vi "Async.vi"() -> ()   [LabVIEW 2012, in "Waveform Data Logger Engine.lvlib"]
uses:
  Waveform Data Logger Engine.lvlib
  Types/RT Data.ctl
  <vilib>/NI Veristand/Custom Device API/Custom Device Item Ref.ctl
  Types/Inline Waveform Info.ctl
  <vilib>/NI Veristand/Custom Device API/Waveform Data Reference.ctl
  Classes/Waveforms/Waveform Receive/Associated Log.ctl
  <vilib>/NI Veristand/Custom Device API/Custom Device Waveform DataType.ctl
  Types/Channels.ctl
  <vilib>/NI Veristand/Custom Device API/Block Data Reference.ctl
  <vilib>/NI Veristand/Custom Device API/Data Reference.ctl
  Types/System Time.ctl
  Types/Inline Waveform Log Info.ctl
  Shared/Classes/Log File Specifications/Waveform TDMS Log File Specification/Waveform TDMS Log File Specification.lvclass
  Classes/Triggers/Trigger/Trigger.lvclass
  Types/Inline Log Waveform.ctl
  Types/Trigger Settings.ctl
  Types/Log Status.ctl
  Types/Channel.ctl
  Types/Communication.ctl
  Types/Async Status.ctl
  Types/Async State.ctl
  <vilib>/NI Veristand/Custom Device Waveform API/Communication Properties.ctl
  Types/Trigger Event Data.ctl
  Types/Trigger Received.ctl
  Types/New File Event Data.ctl
  Types/Log Queues.ctl
  <vilib>/NI Veristand/Custom Device Waveform API/Waveform Session.lvclass/Waveform Session.ctl
  <vilib>/NI Veristand/Custom Device Waveform API/Multiple Waveforms Read (DBL)/Multiple Waveforms Read (DBL).lvclass/Multiple Waveforms Read (DBL).ctl
  <vilib>/NI Veristand/Custom Device Waveform API/Internal Comm Classes/WPL Comm/WPL Comm (1D DBL)/WPL Comm (1D DBL).lvclass/WPL Comm (1D DBL).ctl
  Classes/Waveforms/Utilities/Reference Dictionary/Reference Dictionary.lvclass/Reference Dictionary.ctl
  Classes/Waveforms/Waveform Receive/Waveform Receive.lvclass/Waveform Receive.ctl
  Classes/Waveforms/Waveform Log/Waveform Log.lvclass/Waveform Log.ctl
  Classes/Logs/Segmented Logs/Segmented Log/Segmented Log.lvclass/Segmented Log.ctl
  Shared/Classes/Log File Specifications/Log File Specification/Log File Specification.lvclass/Log File Specification.ctl
  Shared/Classes/Log File Specifications/Waveform TDMS Log File Specification/Waveform TDMS Log File Specification.lvclass/Waveform TDMS Log File Specification.ctl
  Classes/Logs/Log Files/Log File/Log File.lvclass/Log File.ctl
  Classes/Logs/Log Files/TDMS Log File/TDMS Log File.lvclass/TDMS Log File.ctl
  Classes/Logs/Log Files/Text Log File/Text Log File.lvclass/Text Log File.ctl
  Classes/Logs/Segmented Logs/Footprint Segmented Log/Footprint Segmented Log.lvclass/Footprint Segmented Log.ctl
  Classes/Logs/Segmented Logs/Time Segmented Log/Time Segmented Log.lvclass/Time Segmented Log.ctl
  Classes/Waveforms/Buffer/Waveform Buffer/Waveform Buffer.lvclass/Waveform Buffer.ctl
  Classes/Waveforms/Buffer/DBL Waveform Buffer/DBL Waveform Buffer.lvclass/DBL Waveform Buffer.ctl
  Types/Check File Loop Cmd.ctl
  <vilib>/NI Veristand/Custom Device Waveform API/NI VeriStand - Read Waveform(s).vi
  <vilib>/NI Veristand/Custom Device Waveform API/Multiple Waveforms Read (DBL)/NI VeriStand - Read Multiple Waveforms (DBL).vi
  Classes/Waveforms/Utilities/Reference Dictionary/Lookup (Wfm Data Ref).vi
  Classes/Waveforms/Waveform Log/Write Current Waveform to Log Instances.vi
  Classes/Waveforms/Waveform Log/Update Missed Samples.vi
  Classes/Waveforms/Waveform Receive/Check Missed Samples.vi
  Classes/Waveforms/Buffer/Waveform Buffer/Write Waveform to Buffer (DBL).vi
  Classes/Waveforms/Buffer/Waveform Buffer/Set dt.vi
  Classes/Waveforms/Waveform Receive/Get dt.vi
  Classes/Waveforms/Waveform Receive/Check For DBL Equality.vi
  Classes/Waveforms/Buffer/Waveform Buffer/Get Segments in Range.vi
  Classes/Waveforms/Buffer/Waveform Buffer/Read Waveform Segment (DBL).vi
  Classes/Waveforms/Waveform Log/Write to Waveform Log Instance.vi
  Classes/Waveforms/Waveform Log/Update Log Status.vi
  <vilib>/NI Veristand/Custom Device Waveform API/Internal Comm Classes/WPL Comm/WPL Comm (1D DBL)/Comm_read 1d dbl.vi
  <vilib>/NI Veristand/Custom Device Waveform API/Check Opened.vi
  Classes/Waveforms/Waveform Log/Get Waveform In Range.vi
  Classes/Waveforms/Buffer/DBL Waveform Buffer/DBL Write to Buffer.vi
  Classes/Waveforms/Buffer/Waveform Buffer/Update Current Segment.vi
  Classes/Waveforms/Buffer/Waveform Buffer/Check New Segment.vi
  Classes/Waveforms/Buffer/Waveform Buffer/Update Waveform Segments.vi
  Classes/Waveforms/Buffer/Waveform Buffer/Resize Buffer.vi
  Classes/Waveforms/Buffer/Waveform Buffer/Shift Point by Time.vi
  Classes/Waveforms/Buffer/Waveform Buffer/Split Divided Segment.vi
  Classes/Waveforms/Buffer/DBL Waveform Buffer/DBL Read from Buffer.vi
  Classes/Logs/Segmented Logs/Segmented Log/Write Waveform to Log File Instance.vi
  <vilib>/NI Veristand/Custom Device Waveform API/Internal Comm Classes/WPL Comm/Convert Q Error to Shutdown Error.vi
  Classes/Waveforms/Buffer/Waveform Buffer/Get Current Buffer Index.vi
  Classes/Waveforms/Buffer/Waveform Buffer/Get Buffer Length.vi
  Classes/Waveforms/Buffer/Waveform Buffer/Shift Point by Samples.vi
  Classes/Waveforms/Buffer/DBL Waveform Buffer/DBL Resize Buffer.vi
  Shared/Classes/Log File Specifications/Log File Specification/Get Log Specification Type.vi
  Shared/Classes/Log File Specifications/Waveform TDMS Log File Specification/Get Current Group.vi
  Classes/Logs/Log Files/Log File/Get Log File Type.vi
  Classes/Logs/Log Files/Log File/Write Channel to Log File.vi
  Classes/Logs/Log Files/TDMS Log File/Set TDMS Channel Property.vi
  Classes/Logs/Log Files/TDMS Log File/Copy Channel Properties.vi
  Classes/Logs/Segmented Logs/Segmented Log/Check Close File.vi
  Classes/Logs/Segmented Logs/Segmented Log/Check Open File.vi
  Classes/Logs/Log Files/TDMS Log File/Write Channel to TDMS Log File.vi
  Classes/Logs/Log Files/Text Log File/Write Channel to Text Log File.vi
  Classes/Logs/Segmented Logs/Segmented Log/Close Log File Instance.vi
  Classes/Logs/Segmented Logs/Segmented Log/Segment Log File.vi
  Classes/Logs/Segmented Logs/Segmented Log/Open Log File Instance.vi
  Classes/Logs/Log Files/Log File/Close Log File.vi
  Classes/Logs/Segmented Logs/Segmented Log/Make File Read-Only.vi
  Classes/Logs/Segmented Logs/Segmented Log/On Segmented Log Complete.vi
  Classes/Logs/Segmented Logs/Segmented Log/On File Close.vi
  Classes/Logs/Segmented Logs/Footprint Segmented Log/Segment Log File (Footprint).vi
  Classes/Logs/Segmented Logs/Time Segmented Log/Segment Log File (Time).vi
  Shared/Classes/Log File Specifications/Log File Specification/Open Log File.vi
  Shared/Classes/Log File Specifications/Log File Specification/Set Path Tag.vi
  Classes/Logs/Segmented Logs/Segmented Log/On File Open.vi
  Shared/Classes/Log File Specifications/Log File Specification/Set Filename Offset.vi
  Classes/Logs/Log Files/TDMS Log File/Close TDMS Log File.vi
  Classes/Logs/Log Files/Text Log File/Close Text Log File.vi
  Classes/Logs/Segmented Logs/Segmented Log/Get Current Log File Instance.vi
  Classes/Logs/Log Files/Log File/Get File Size.vi
  Classes/Logs/Log Files/Log File/Get Start Time.vi
  Shared/Classes/Log File Specifications/Log File Specification/Build File Path.vi
  Shared/Classes/Log File Specifications/Log File Specification/Resolve File Conflicts.vi
  <vilib>/Utility/error.llb/Error Cluster From Error Code.vi
  Classes/Waveforms/Waveform Log/Check Instance Done.vi
  Shared/Classes/Log File Specifications/Log File Specification/Initialize Log File.vi
  <vilib>/Utility/libraryn.llb/Check if File or Folder Exists.vi
  <vilib>/Utility/libraryn.llb/Get File Extension.vi
  <vilib>/Utility/libraryn.llb/Create Directory Recursive.vi
  <userlib>/_OpenG.lib/error/error.llb/Filter Error Codes (Array)__ogtk.vi
  <vilib>/NI Veristand/Custom Device Tools/Custom Device Utility Library/NI VeriStand - Print Debug String.vi
  <vilib>/Utility/error.llb/Simple Error Handler.vi
  Classes/Waveforms/Waveform Receive/Waveform Receive.lvclass
  Classes/Logs/Log Files/Log File/Log File.lvclass
  Classes/Logs/Log Files/TDMS Log File/TDMS Log File.lvclass
  Classes/Logs/Log Files/Text Log File/Text Log File.lvclass
  Classes/Logs/Segmented Logs/Footprint Segmented Log/Footprint Segmented Log.lvclass
  Classes/Logs/Segmented Logs/Time Segmented Log/Time Segmented Log.lvclass
  Classes/Waveforms/Buffer/DBL Waveform Buffer/DBL Waveform Buffer.lvclass
  Classes/Waveforms/Buffer/CDB Waveform Buffer/CDB Waveform Buffer.lvclass
  <vilib>/NI VeriStand/Custom Device Waveform API/NI_VS Custom Device Waveform API.lvlib
  Classes/Waveforms/Waveform Log/Waveform Log.lvclass
  <vilib>/NI Veristand/Custom Device Waveform API/Multiple Waveforms Read (CDB)/NI VeriStand - Open Multiple Waveforms Read Session (CDB).vi
  <vilib>/NI Veristand/Custom Device Waveform API/Multiple Waveforms Read (CDB)/Multiple Waveforms Read (CDB).lvclass
  <vilib>/NI Veristand/Custom Device API/Custom Device API.lvlib
panel:
  in  "Async Input":T1={"Device Ref"=18446744073709551615, "Waveforms"=[], "Channels"={"Command Chan Refs"=[], "Command Data Refs"=[], "Command Values"=[], "Status Chan Refs"=[], "Status Data Refs"=[], "Status Values"=[], "System Time"={"System Time"=timestamp(0 s since 1904-01-01), "Data Reference"=0, "Absolute Time Channel Data Ref"=0, "Get Date-Time Channel Data Ref"=0}, "Trigger Chan Refs"=[], "Trigger Data Refs"=[], "Trigger Values"=[]}, "Waveform Logs"=[], "Communication"={"Async Status"=refnum, "Wfm Comm Properties"={"WPL"={"Custom Queue Size"=1, "Use Custom Queue Size?"=FALSE}}, "Shutdown Event"=refnum, "Trigger Event"=refnum, "New File Event"=refnum, "Log Queues"=[], "Async VI Ref"=refnum}, "error"={"status"=FALSE, "code"=0, "source"=""}} {"Device Ref" format="%.0x"; "Channels"."Trigger Data Refs"."Data Reference" format="%.0x"; "Channels"."Trigger Chan Refs" format="%.0x"; "Channels"."System Time"."Get Date-Time Channel Data Ref" format="%.0x"; "Channels"."System Time"."Absolute Time Channel Data Ref" format="%.0x"; "Channels"."System Time"."Channel Data Reference" format="%.0x"; "Channels"."Status Data Refs"."Data Reference" format="%.0x"; "Channels"."Command Data Refs"."Data Reference" format="%.0x"; "Channels"."Status Chan Refs" format="%.0x"; "Channels"."Command Chan Refs" format="%.0x"; "Waveforms"."Waveform Ref in" format="%.0x"; "Waveform Logs"."Node ID" format="%.0x"; "Waveform Logs"."TDMS Error Code"."Data Ref" format="%.0x"; "Waveform Logs"."Missed Samples"."Data Ref" format="%.0x"; "Waveform Logs"."File Status"."Data Ref" format="%.0x"; "Waveform Logs"."Start New File"."Data Ref" format="%.0x"; "Waveform Logs"."Logging Enabled"."Data Ref" format="%.0x"; "Waveform Logs"."Stop Trigger"."Node Data Ref" format="%.0x"; "Waveform Logs"."Stop Trigger"."Node ID" format="%.0x"; "Waveform Logs"."Start Trigger"."Node Data Ref" format="%.0x"; "Waveform Logs"."Start Trigger"."Node ID" format="%.0x"}
  out "error out":errorcluster
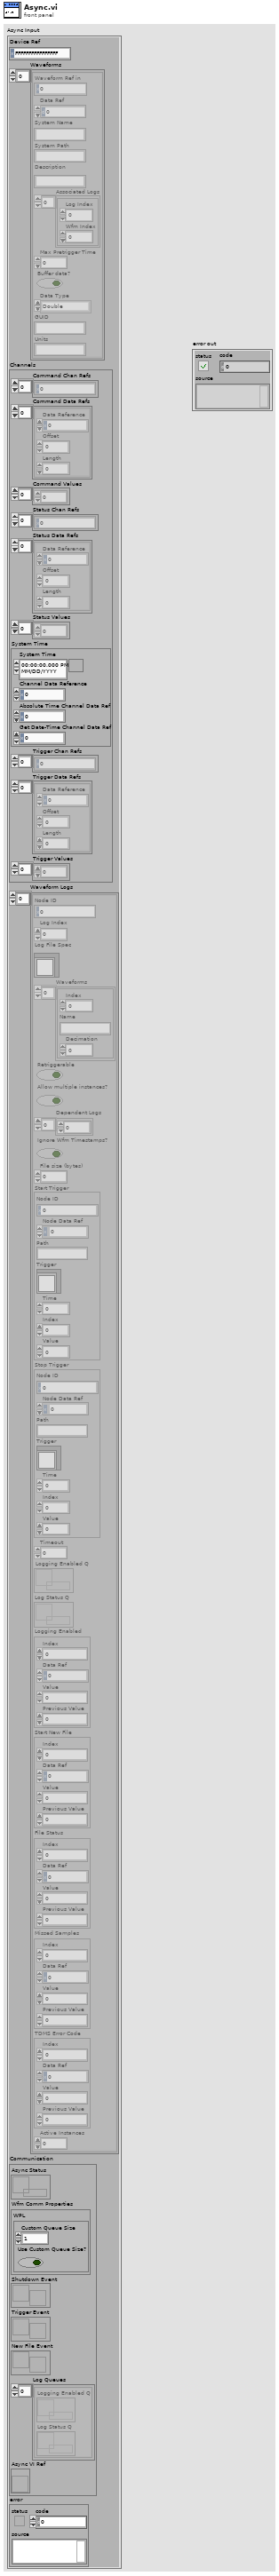
[diagram p1: front panel]
types:
  T1 = typedef "Waveform Data Logger Engine.lvlib/RT Data.ctl" = cluster{"Device Ref":T2, "Waveforms":T3[], "Channels":T7, "Waveform Logs":T11[], "Communication":T15, "error":errorcluster}
  T2 = typedef "Custom Device API.lvlib/Custom Device Item Ref.ctl" = u64
  T3 = typedef "Waveform Data Logger Engine.lvlib/Inline Waveform Info.ctl" = cluster{"Waveform Ref in":T2, "Data Ref":T4, "System Name":string, "System Path":string, "Description":string, "Associated Logs":T5[], "Max Pretrigger Time":dbl, "Buffer data?":bool, "Data Type":T6, "GUID":string, "Units":string}
  T4 = typedef "Custom Device API.lvlib/Waveform Data Reference.ctl" = i32
  T5 = typedef "Waveform Data Logger Engine.lvlib/Waveform Receive.lvclass/Associated Log.ctl" = cluster{"Log Index":i32, "Wfm Index":i32}
  T6 = typedef "Custom Device API.lvlib/Custom Device Waveform DataType.ctl" = enum16{"Double", "Complex Double"}
  T7 = typedef "Waveform Data Logger Engine.lvlib/Channels.ctl" = cluster{"Command Chan Refs":T2[], "Command Data Refs":T8[], "Command Values":dbl[], "Status Chan Refs":T2[], "Status Data Refs":T8[], "Status Values":dbl[], "System Time":T10, "Trigger Chan Refs":T2[], "Trigger Data Refs":T8[], "Trigger Values":dbl[]}
  T8 = typedef "Custom Device API.lvlib/Block Data Reference.ctl" = cluster{"Data Reference":T9, "Offset":i32, "Length":i32}
  T9 = typedef "Custom Device API.lvlib/Data Reference.ctl" = i32
  T10 = typedef "Waveform Data Logger Engine.lvlib/System Time.ctl" = cluster{"System Time":timestamp, "Data Reference":T9, "Absolute Time Channel Data Ref":T9, "Get Date-Time Channel Data Ref":T9}
  T11 = typedef "Waveform Data Logger Engine.lvlib/Inline Waveform Log Info.ctl" = cluster{"Node ID":T2, "Log Index":i32, "Log File Spec":refnum<class "Waveform TDMS Log File Specification.lvclass">, "Waveforms":T12[], "Retriggerable":bool, "Allow multiple instances?":bool, "Dependent Logs":i32[], "Ignore Wfm Timestamps?":bool, "File size (bytes)":i64, "Start Trigger":T13, "Stop Trigger":T13, "Timeout":dbl, "Logging Enabled Q":refnum<queue>, "Log Status Q":refnum<queue>, "Logging Enabled":T14, "Start New File":T14, "File Status":T14, "Missed Samples":T14, "TDMS Error Code":T14, "Active Instances":i32}
  T12 = typedef "Waveform Data Logger Engine.lvlib/Inline Log Waveform.ctl" = cluster{"Index":i32, "Name":string, "Decimation":u32}
  T13 = typedef "Waveform Data Logger Engine.lvlib/Trigger Settings.ctl" = cluster{"Node ID":T2, "Node Data Ref":i32, "Path":string, "Trigger":refnum<class "Trigger.lvclass">, "Time":dbl, "Index":i32, "Value":dbl}
  T14 = typedef "Waveform Data Logger Engine.lvlib/Channel.ctl" = cluster{"Index":i32, "Data Ref":T9, "Value":dbl, "Previous Value":dbl}
  T15 = typedef "Waveform Data Logger Engine.lvlib/Communication.ctl" = cluster{"Async Status":refnum<queue>, "Wfm Comm Properties":T16, "Shutdown Event":refnum<user-event>, "Trigger Event":refnum<user-event>, "New File Event":refnum<user-event>, "Log Queues":T17[], "Async VI Ref":refnum<vi>}
  T16 = typedef "NI_VS Custom Device Waveform API.lvlib/Communication Properties.ctl" = cluster{"WPL":cluster{"Custom Queue Size":i32, "Use Custom Queue Size?":bool}}
  T17 = typedef "Waveform Data Logger Engine.lvlib/Log Queues.ctl" = cluster{"Logging Enabled Q":refnum<queue>, "Log Status Q":refnum<queue>}
  T18 = typedef "Waveform Data Logger Engine.lvlib/Async State.ctl" = enum16{"Not running", "Initializing", "Running", "Stopped"}
  T19 = typedef "Waveform Data Logger Engine.lvlib/Async Data.ctl" = cluster{"Wfm Read Session (DBL)":refnum<class "Multiple Waveforms Read (DBL).lvclass">, "DBL Wfm Acq Data":T20, "Wfm Logs":refnum<data-value>[], "Async Communication":T21}
  T20 = typedef "Waveform Data Logger Engine.lvlib/Wfm Acq Data.ctl" = cluster{"Wfm Ref Dictionary":refnum<class "Reference Dictionary.lvclass">, "Received Wfms":refnum<data-value>[]}
  T21 = typedef "Waveform Data Logger Engine.lvlib/Async Communication.ctl" = cluster{"Shutdown":refnum<user-event>, "Check File Loop Cmd":refnum<queue>}
  T22 = typedef "Waveform Data Logger Engine.lvlib/Check File Loop Cmd.ctl" = enum16{"None", "Stop"}
  T23 = typedef "Trigger Received.ctl" = enum16{"None", "Start", "Stop", "Both", "Disable"}
  T24 = typedef "NI_VS Custom Device Waveform API.lvlib/Waveform properties.ctl" = cluster{"Data reference":T4, "t0 at start":timestamp, "dt":dbl, "offset from start (samples)":u64}
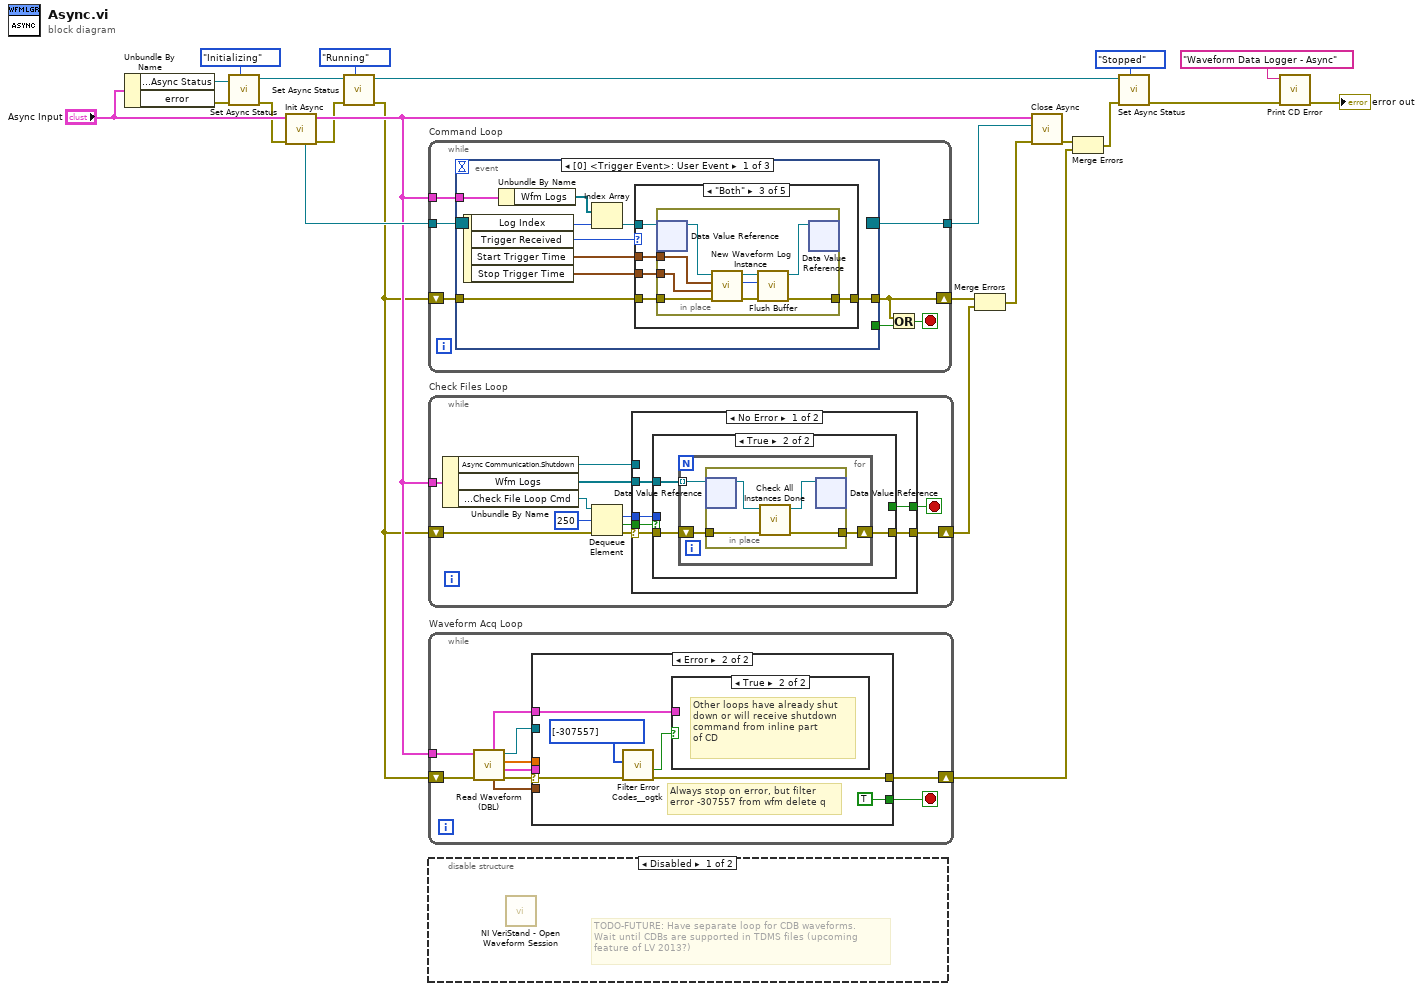
[diagram p0: block diagram]
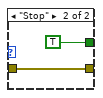
[diagram p4: hidden frame]
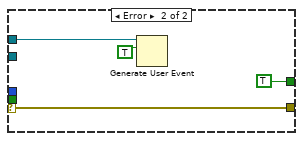
[diagram p5: hidden frame]
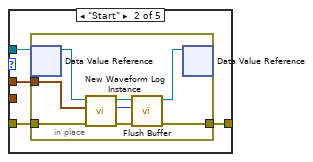
[diagram p7: hidden frame]
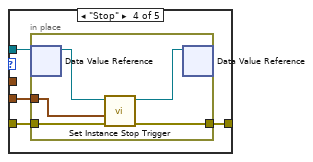
[diagram p8: hidden frame]
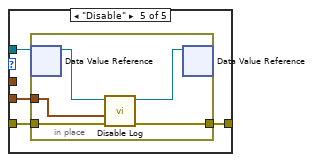
[diagram p9: hidden frame]
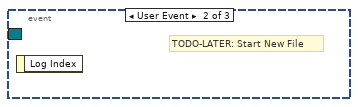
[diagram p10: hidden frame]
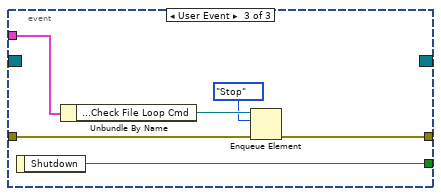
[diagram p11: hidden frame]
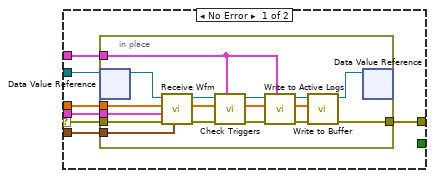
[diagram p12: hidden frame]
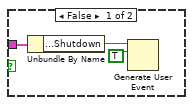
[diagram p13: hidden frame]
diagram:
  n1 = Unbundle By Name("Async Input") -> ("Communication.Async Status"=w14:refnum<queue>, "error"=w8:errorcluster)
  n2 = call "Set Async Status.vi"("State"=Async_State."Initializing", "error in (no error)"=w8, "Async Status in"=w14) -> ("error out"=w7:errorcluster, "Async Status out"=w10:refnum<queue>)  [unwired: 7 in]
  n3 = call "Init Async.vi"("error in (no error)"=w7, "Async Input"="Async Input") -> ("error out"=w11:errorcluster, "Async Data"=w21:T19, "Event Registration"=w22:refnum<event-registration>)  [unwired: 7 in]
  n4 = call "Set Async Status.vi"("State"=Async_State."Running", "error in (no error)"=w11, "Async Status in"=w10) -> ("error out"=w9:errorcluster, "Async Status out"=w5:refnum<queue>)  [unwired: 7 in]
  n5 = while "Command Loop" {
    tunnel: w22 -> [w30]
    tunnel: w21 -> [w29]
    shift-right: [w25] -> w20
    shift-left: w9 -> [w28]
    tunnel: [w24] -> w16
    stop <- w27 stop-if-true
    n6 = event shown="[0] <Trigger Event>: User Event" {
      selector: w30 -> [_ _ _]
      dyn-events: [_ _ _] -> w24
      timeout: _ -> [_ _ _]
      tunnel: w29 -> [w39 _ w89]
      tunnel: w28 -> [w36 _ w88]
      tunnel: [_ _ w90] -> w26
      tunnel: [w35 _ w85] -> w25
      event User Event {
        n7 = event-data() -> ("Log Index"=w34:i32, "Trigger Received"=w31:T23, "Start Trigger Time"=w33:timestamp, "Stop Trigger Time"=w32:timestamp)  [unwired: 1 in]
        n8 = Unbundle By Name(w39) -> ("Wfm Logs"=w38:refnum<data-value>[])
        n9 = Index Array(array=w38, index=w34) -> (element=w37:refnum<data-value>)
        n10 = case shown="\"Both\"" w31 {
          tunnel: w37 -> [_ w44 w57 w70 w78]
          tunnel: w33 -> [_ w43 w56 _ _]
          tunnel: w32 -> [_ _ w55 w69 w77]
          tunnel: w36 -> [w40 w42 w54 w68 w79]
          tunnel: [w40 w41 w53 w67 w76] -> w35
          frame "None", Default {
            # "TODO-LATER: Throw Error.\nUnexpected Case"
          }
          frame "Start" {
            n11 = in-place {
              in-place-border: w43 -> [w51]
              in-place-border: w42 -> [w48]
              in-place-border: [w47] -> w41
              n12 = in-place-dvr #1(w44) -> (w52:refnum<class "Waveform Log.lvclass">)  [unwired: 1 out]
              n13 = call "New Waveform Log Instance.vi"("error in (no error)"=w48, "Start Trigger Time"=w51, "Waveform Log in"=w52) -> ("error out"=w49:errorcluster, "Wfm Log Instance Index"=w45:i32, "Waveform Log out"=w50:refnum<class "Waveform Log.lvclass">)  [unwired: 6 in]
              n14 = call "Flush Buffer.vi"("error in (no error)"=w49, "Wfm Log Instance Index"=w45, "Waveform Log in"=w50) -> ("error out"=w47:errorcluster, "Waveform Log out"=w46:refnum<class "Waveform Log.lvclass">)  [unwired: 7 in]
              n15 = in-place-dvr #1(w46) -> ()  [unwired: 2 out]
            }
          }
          frame "Both" {
            n16 = in-place {
              in-place-border: w56 -> [w65]
              in-place-border: w55 -> [w64]
              in-place-border: w54 -> [w61]
              in-place-border: [w60] -> w53
              n17 = in-place-dvr #2(w57) -> (w66:refnum<class "Waveform Log.lvclass">)  [unwired: 1 out]
              n18 = call "New Waveform Log Instance.vi"("error in (no error)"=w61, "Stop Trigger Time (optional)"=w64, "Start Trigger Time"=w65, "Waveform Log in"=w66) -> ("error out"=w62:errorcluster, "Wfm Log Instance Index"=w58:i32, "Waveform Log out"=w63:refnum<class "Waveform Log.lvclass">)  [unwired: 5 in]
              n19 = call "Flush Buffer.vi"("error in (no error)"=w62, "Wfm Log Instance Index"=w58, "Waveform Log in"=w63) -> ("error out"=w60:errorcluster, "Waveform Log out"=w59:refnum<class "Waveform Log.lvclass">)  [unwired: 7 in]
              n20 = in-place-dvr #2(w59) -> ()  [unwired: 2 out]
            }
          }
          frame "Stop" {
            n21 = in-place {
              in-place-border: w69 -> [w72]
              in-place-border: w68 -> [w74]
              in-place-border: [w73] -> w67
              n22 = in-place-dvr #3(w70) -> (w75:refnum<class "Waveform Log.lvclass">)  [unwired: 1 out]
              n23 = call "Set Instance Stop Trigger.vi"("error in (no error)"=w74, "Stop Trigger Time"=w72, "Waveform Log in"=w75) -> ("error out"=w73:errorcluster, "Waveform Log out"=w71:refnum<class "Waveform Log.lvclass">)  [unwired: 7 in]
              n24 = in-place-dvr #3(w71) -> ()  [unwired: 2 out]
            }
          }
          frame "Disable" {
            n25 = in-place {
              in-place-border: w77 -> [w81]
              in-place-border: w79 -> [w83]
              in-place-border: [w82] -> w76
              n26 = in-place-dvr #4(w78) -> (w84:refnum<class "Waveform Log.lvclass">)  [unwired: 1 out]
              n27 = call "Disable Log.vi"("error in (no error)"=w83, "Stop Trigger Time"=w81, "Waveform Log in"=w84) -> ("error out"=w82:errorcluster, "Waveform Log out"=w80:refnum<class "Waveform Log.lvclass">)  [unwired: 7 in]
              n28 = in-place-dvr #4(w80) -> ()  [unwired: 2 out]
            }
          }
        }
      }
      event User Event {
        # "TODO-LATER: Start New File"
        n29 = event-data() -> ()  [unwired: 1 in, 1 out]
      }
      event User Event {
        n30 = event-data() -> ("Shutdown"=w90:bool)  [unwired: 1 in]
        n31 = Unbundle By Name(w89) -> ("Async Communication.Check File Loop Cmd"=w87:refnum<queue>)
        n32 = Enqueue Element(queue=w87, element=Check_File_Loop_Cmd."Stop", error in (no error)=w88) -> (error out=w85:errorcluster)  [unwired: 1 in, 2 out]
      }
    }
    n33 = Or(x=w25, y=w26) -> (x .or. y?=w27:bool)
  }
  n34 = while "Check Files Loop" {
    tunnel: w21 -> [w95]
    shift-right: [w101] -> w19
    shift-left: w9 -> [w96]
    stop <- w100 stop-if-true
    n35 = Unbundle By Name(w95) -> ("Async Communication.Shutdown"=w91:refnum<user-event>, "Wfm Logs"=w97:refnum<data-value>[], "Async Communication.Check File Loop Cmd"=w98:refnum<queue>)
    n36 = Dequeue Element(queue=w98, timeout in ms (-1)=250, error in (no error)=w96) -> (element=w92:T22, timed out?=w94:bool, error out=w93:errorcluster)  [unwired: 1 out]
    n37 = case shown="No Error" w93 {
      selector: w93 -> [w103 w128]
      tunnel: [w107 w128] -> w101
      tunnel: [w106 TRUE] -> w100
      tunnel: w97 -> [w105 _]
      tunnel: w94 -> [w104 _]
      tunnel: w92 -> [w102 _]
      tunnel: w91 -> [_ w125]
      frame No Error {
        n38 = case shown="True" w104 {
          tunnel: [w111 w115] -> w107
          tunnel: [w108 _] -> w106
          tunnel: w105 -> [_ w117]
          tunnel: w103 -> [w110 w116]
          tunnel: w102 -> [w109 _]
          frame False {
            n39 = case shown="\"None\", Default" w109 {
              tunnel: [w112 w114] -> w111
              tunnel: w110 -> [w112 w114]
              tunnel: [_ TRUE] -> w108
              frame "None", Default {
              }
              frame "Stop" {
              }
            }
          }
          frame True {
            n40 = for {
              tunnel: w117 -> [w120] mode=indexing
              shift-right: [w118] -> w115
              shift-left: w116 -> [w119]
              n41 = in-place {
                in-place-border: w119 -> [w123]
                in-place-border: [w122] -> w118
                n42 = in-place-dvr #5(w120) -> (w124:refnum<class "Waveform Log.lvclass">)  [unwired: 1 out]
                n43 = call "Check All Instances Done.vi"("error in (no error)"=w123, "Waveform Log in"=w124) -> ("error out"=w122:errorcluster, "Waveform Log out"=w121:refnum<class "Waveform Log.lvclass">)  [unwired: 8 in]
                n44 = in-place-dvr #5(w121) -> ()  [unwired: 2 out]
              }
            }
          }
        }
      }
      frame Error {
        n45 = Generate User Event(user event=w125, event data cluster=TRUE ("event data")) -> ()  [unwired: 1 in, 2 out]
      }
    }
  }
  n46 = while "Waveform Acq Loop" {
    tunnel: w21 -> [w132]
    shift-right: [w130] -> w17
    shift-left: w9 -> [w135]
    stop <- w129 stop-if-true
    n47 = call "Read Waveform (DBL).vi"("error in (no error)"=w135, "Async Data in"=w132) -> ("error out"=w138:errorcluster, "Properties"=w137:T24, "Data"=w136:dbl[], "Received Wfm"=w134:refnum<data-value>, "Receive Time"=w133:timestamp, "Async Data out"=w131:T19)  [unwired: 4 in]
    n48 = case shown="Error" w138 {
      selector: w138 -> [w145 w166]
      tunnel: w137 -> [w144 _]
      tunnel: w136 -> [w142 _]
      tunnel: w134 -> [w143 _]
      tunnel: w133 -> [w141 _]
      tunnel: w131 -> [w140 w164]
      tunnel: [w139 w163] -> w130
      tunnel: [_ TRUE] -> w129
      frame No Error {
        n49 = in-place {
          in-place-border: w145 -> [w155]
          in-place-border: w144 -> [w152]
          in-place-border: w142 -> [w151]
          in-place-border: w141 -> [w153]
          in-place-border: w140 -> [w146]
          in-place-border: [w147] -> w139
          n50 = in-place-dvr #6(w143) -> (w150:refnum<class "Waveform Receive.lvclass">)  [unwired: 1 out]
          n51 = call "Receive Wfm.vi"("Receive Time"=w153, "error in (no error)"=w155, "Wfm Properties"=w152, "Data in"=w151, "Waveform Receive in"=w150) -> ("error out"=w154:errorcluster, "Data out"=w148:dbl[], "Waveform Receive out"=w149:refnum<class "Waveform Receive.lvclass">)  [unwired: 4 in]
          n52 = call "Check Triggers.vi"("Async Data in"=w146, "error in (no error)"=w154, "Data in"=w148, "Waveform Receive in"=w149) -> ("error out"=w162:errorcluster, "Data out"=w158:dbl[], "Waveform Receive out"=w159:refnum<class "Waveform Receive.lvclass">)  [unwired: 5 in]
          n53 = call "Write to Active Logs.vi"("Async Data in"=w146, "error in (no error)"=w162, "Data in"=w158, "Waveform Receive in"=w159) -> ("error out"=w161:errorcluster, "Data out"=w156:dbl[], "Waveform Receive out"=w157:refnum<class "Waveform Receive.lvclass">)  [unwired: 5 in]
          n54 = call "Write to Buffer.vi"("error in (no error)"=w161, "Data in"=w156, "Waveform Receive in"=w157) -> ("error out"=w147:errorcluster, "Waveform Receive out"=w160:refnum<class "Waveform Receive.lvclass">)  [unwired: 7 in]
          n55 = in-place-dvr #6(w160) -> ()  [unwired: 2 out]
        }
      }
      frame Error {
        # "Always stop on error, but filter\nerror -307557 from wfm delete q"
        n56 = call-poly <userlib>:"Filter Error Codes__ogtk.vi"("Error In"=w166, "Error Codes to Filter"=i32[] [-307557]) -> ("Error Out"=w163:errorcluster, "Error Filtered?"=w165:bool)  [unwired: 7 in, 1 out]
        n57 = case shown="True" w165 {
          tunnel: w164 -> [w170 _]
          frame False {
            n58 = Unbundle By Name(w170) -> ("Async Communication.Shutdown"=w171:refnum<user-event>)
            n59 = Generate User Event(user event=w171, event data cluster=TRUE ("event data")) -> ()  [unwired: 1 in, 2 out]
          }
          frame True {
            # "Other loops have already shut\ndown or will receive shutdown\ncommand from inline part\nof CD"
          }
        }
      }
    }
  }
  n60 = disable-structure shown="Disabled" {
    frame Disabled {
      # "TODO-FUTURE: Have separate loop for CDB waveforms.\nWait until CDBs are supported in TDMS files (upcoming\nfeature of LV 2013?)"
      n61 = call-poly <vilib>:"NI VeriStand - Open Waveform Session.vi"() -> ()  [unwired: 10 in, 2 out]
    }
    frame Enabled {
    }
  }
  n62 = Merge Errors(w20, w19) -> (w23:errorcluster)
  n63 = call "Close Async.vi"("error in (no error)"=w23, "Event Registration"=w16, "Async Data"=w21) -> ("error out"=w18:errorcluster)  [unwired: 8 in]
  n64 = Merge Errors(w18, w17) -> (w4:errorcluster)
  n65 = call "Set Async Status.vi"("State"=Async_State."Stopped", "error in (no error)"=w4, "Async Status in"=w5) -> ("error out"=w2:errorcluster)  [unwired: 7 in, 1 out]
  n66 = call "Print CD Error.vi"("error in"=w2, "Your code's public name"="Waveform Data Logger - Async") -> ("error out"=→"error out":errorcluster)  [unwired: 8 in]
